vi "Write Device ID Type.vi"(8 "error in":errorcluster, 10 "device ID type":T1=1 items=["None"=0, "Basic Stream"=1, "Regular Stream"=2, "Extended Stream"=3, "Basic Stream/Individual"=129, "Regular Stream/Individual"=130, "Extended Stream/Individual"=131], 11 "device data model in":refnum<class "Standard Data Model.lvclass">) -> (0 "error out":errorcluster, 3 "device data model out":refnum<class "Standard Data Model.lvclass">)   [LabVIEW 2013, in "Modbus Library - Advance.lvlib" / "Standard Data Model.lvclass"]
doc: "Writes the value of the device ID."
uses:
  Standard Data Model.lvclass
  Data Model/Device ID Type.ctl
  Standard Data Model.lvclass/Standard Data Model.ctl
  Data Model/Device Data Model.lvclass
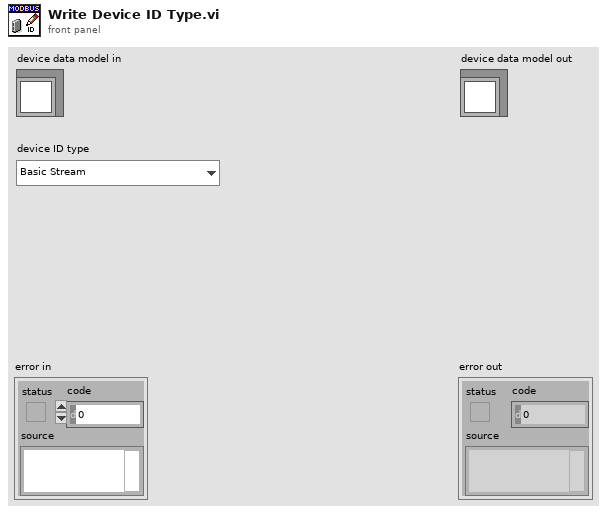
[diagram p1: front panel]
types:
  T1 = typedef "Modbus Library - Advance.lvlib/Device Data Model.lvclass/Device ID Type.ctl" = u8
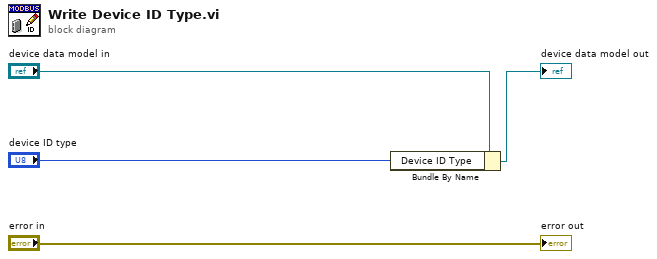
[diagram p0: block diagram]
diagram:
  n1 = Bundle By Name(cluster="device data model in", "Device ID Type"="device ID type") -> (→"device data model out":refnum<class "Standard Data Model.lvclass">)
  "error out" <- "error in"
